vi "Dispose Empty Channels.vi"   [LabVIEW 2020, in "Actor Pub Sub Channels.lvlib"]
uses:
  Actor Pub Sub Channels.lvlib
  Pub Sub Message Channel/Has Receivers.vi
  Pub Sub Message Channel/Pub Sub Message Channel.lvclass
types:
  T1 = enum16{"Nothing", "Get Channel", "Get Or Create Channel", "Close Channel", "Dispose"}
  T2 = map{string, refnum<class "Pub Sub Message Channel.lvclass">}
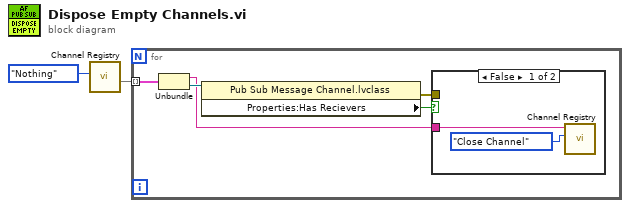
[diagram p0: block diagram]
diagram:
  n1 = call "Channel Registry.vi"("Action"=T1."Nothing") -> ("Registered Channels"=w1:T2)  [unwired: 8 in, 2 out]
  n2 = for {
    tunnel: w1 -> [w7] mode=indexing
    n3 = Unbundle(w7) -> ("Topic"=w3:string, "Pub Sub Message Channel out"=w6:refnum<class "Pub Sub Message Channel.lvclass">)
    n4 = property class="Pub Sub Message Channel.lvclass"(reference=w6) -> (error out=w4:errorcluster, "Properties:Has Recievers"=w5:bool)  [unwired: 1 in, 1 out]
    n5 = case shown="False" w5 {
      tunnel: w4 -> [_ _]
      tunnel: w3 -> [w9 _]
      frame False {
        n6 = call "Channel Registry.vi"("Action"=T1."Close Channel", "Topic"=w9) -> ()  [unwired: 7 in, 3 out]
      }
      frame True {
      }
    }
  }
